vi "Set Output Limits.vi"(7 "Set Limits (T: Voltage)":bool=TRUE, 8 "error in (no error)":errorcluster, 9 "Positive Limit Value (0.0010)":dbl=0.001 format="%^.3e", 10 "Negative Limit Value (-0.0010)":dbl=-0.001 format="%^.3e", 11 "VISA resource name":refnum<visa-resource-name>) -> (0 "error out":errorcluster, 3 "VISA resource name out":refnum<visa-resource-name>)   [LabVIEW 2013, in "Fluke 5XXX Series Multicalibrators.lvlib"]
doc: "This VI sets the maximum permissible output magnitude, negative and positive, for voltage and current, which is saved in the Calibrator non-volatile memory.\n\nThe magnitude of the limit has the following effect on different waveforms:\n\n dc magnitude of limit\n ac (sinewave) magnitude of limit (rms)\n ac (non-sinewave) magnitude of limit x 3 (peak-to-peak)\n ac (with dc offset) magnitude of limit x 2.4 (absolute\n peak) (volts only)\n\nNote:\n\nWhile saving configuration data in the non-volatile memory, a period of about 2 seconds, the Calibrator does not respond to remote commands."
uses:
  Fluke 5XXX Series Multicalibrators.lvlib
panel:
  # "Voltage"
  # "Current"
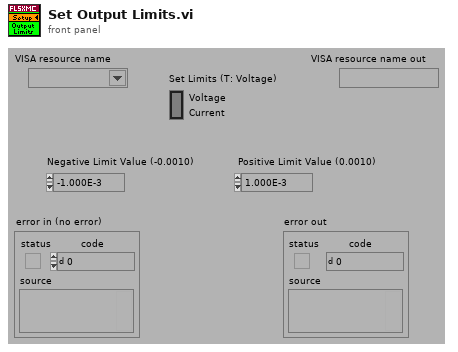
[diagram p1: front panel]
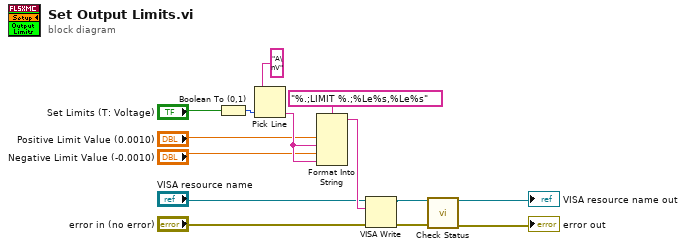
[diagram p0: block diagram]
diagram:
  n1 = Boolean To (0,1)(Boolean="Set Limits (T: Voltage)") -> (0, 1=w11:i16)
  n2 = Pick Line(multi-line string="A\nV", line index=w11) -> (output string=w9:string)  [unwired: 1 in]
  n3 = Format Into String(format string="%.;LIMIT %.;%Le%s,%Le%s", "Positive Limit Value (0.0010)", w9, "Negative Limit Value (-0.0010)", w9) -> (resulting string=w12:string)  [unwired: 2 in, 1 out]
  n4 = VISA Write(VISA resource name="VISA resource name", write buffer=w12, error in (no error)="error in (no error)") -> (VISA resource name out=w14:refnum<visa-resource-name>, error out=w6:errorcluster)  [unwired: 1 out]
  n5 = call "Check Status.vi"("VISA resource name"=w14, "error in (no error)"=w6) -> ("VISA resource name out"=→"VISA resource name out":refnum<visa-resource-name>, "error out"=→"error out":errorcluster)  [unwired: 12 in]
